vi "SHI_MCC_interface.vi"() -> ()   [LabVIEW 2017]
uses:
  <vilib>/httpClient/LabVIEWHTTPClient.lvlib
  <vilib>/httpClient/ClientHandle.ctl
  <vilib>/httpClient/POSTBuffer.vi
  msg7171_linux.llb/send single message.vi
  Type_Defs/Digital_Out.ctl
  Type_Defs/Digital_In_1.ctl
  Type_Defs/Analog_In.ctl
  msg7171_linux.llb/send multiple messages.vi
panel:
  out "Get Params json":string
  out "Get Status json":string
  in  "exit":bool
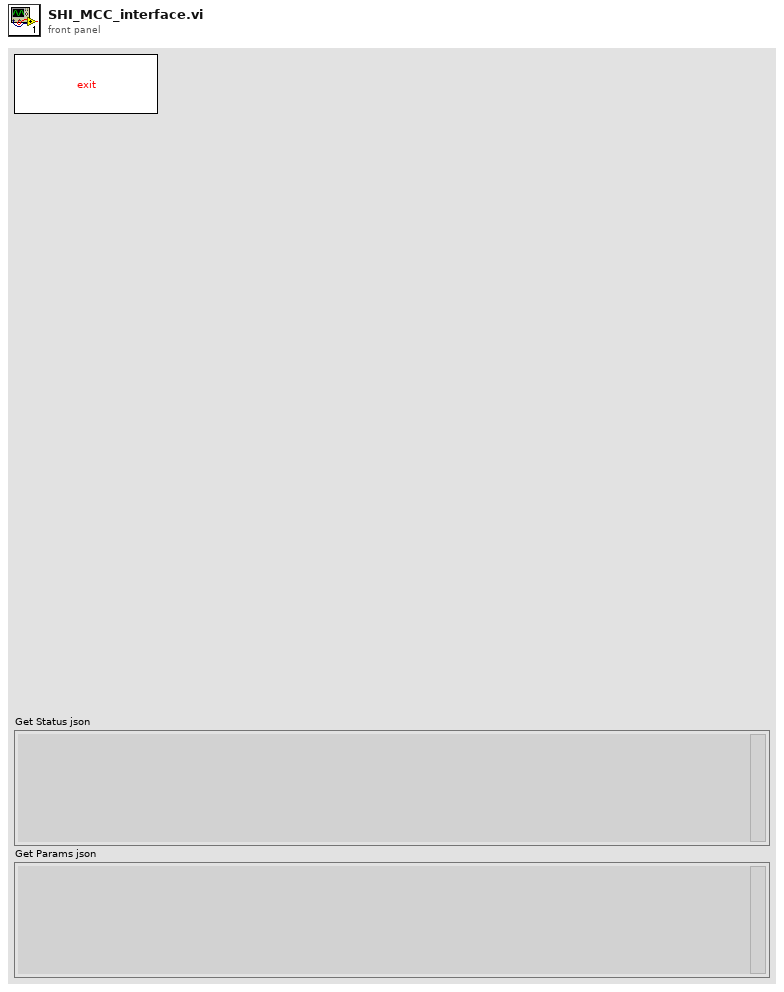
[diagram p1: front panel]
types:
  T1 = typedef "LabVIEWHTTPClient.lvlib/ClientHandle.ctl" = refnum<k1>
  T2 = cluster{"go":bool, "Http session":T1, "URL prefex":string, "Next get param":u32}
  T3 = typedef "Digital_Out.ctl" = cluster{"LN2-P EN":bool, "LN2-S EN":bool, "LN2-Sol EN":bool, "IR Lamp 1":bool, "IR Lamp 2":bool, "IR Lamp 3":bool, "IR Lamp 4":bool, "IR Lamp 5":bool, "IR Lamp 6":bool, "IR Lamp 7":bool, "IR Lamp 8":bool, "IR Lamp 9":bool, "IR Lamp 10":bool, "IR Lamp 11":bool, "IR Lamp 12":bool, "IR Lamp 13":bool, "IR Lamp 14":bool, "IR Lamp 15":bool, "IR Lamp 16":bool, "Heater SSR 1":bool, "Heater SSR 2":bool, "Heater SSR 3":bool, "Heater SSR 4":bool, "Heater SSR 5":bool, "Heater SSR 6":bool, "Heater SSR 7":bool, "Heater SSR 8":bool, "Heater SSR 9":bool, "Heater SSR 10":bool, "Heater SSR 11":bool, "Heater SSR 12":bool, "Heater SSR 13":bool, "Heater SSR 14":bool, "Heater SSR 15":bool, "Heater SSR 16":bool, "Heater SSR 17":bool, "Heater SSR 18":bool, "Heater SSR 19":bool, "Heater SSR 20":bool, "Heater SSR 21":bool, "MCC Power":bool, "MCC2 Power":bool, "RoughP GateValve":bool, "RoughP Start":bool, "CryoP GateValve":bool, "RoughP PurgeGass":bool, "LN2-S Sol":bool, "LN2-P Sol":bool, "CryoP Pwr Relay 1":bool, "CryoP Pwr Relay 2":bool, "RoughP Pwr Relay":bool}
  T4 = typedef "Digital_In_1.ctl" = cluster{"PG-SW-RoughP-Relay 1":bool, "PG-SW-RoughP-Relay 2":bool, "PG-SW-CryoP-Relay 1":bool, "PG-SW-CryoP-Relay 2":bool, "PG-SW-Chamber-Relay 1":bool, "PG-SW-Chamber-Relay 2":bool, "LN2-P-Sol-Open: NC":bool, "LN2-P-Sol-Open: O":bool, "LN2-P-Sol-Closed: NC":bool, "LN2-P-Sol-Closed: O":bool, "LN2-S-Sol-Open: NC":bool, "LN2-S-Sol-Open: O":bool, "LN2-S-Sol-Closed: NC":bool, "LN2-S-Sol-Closed: O":bool, "CryoP-GV-Open: NC":bool, "CryoP-GV-Open: O":bool, "CryoP-GV-Closed: NC":bool, "CryoP-GV-Closed: O":bool, "RoughP-GV-Open":bool, "RoughP-GV-Closed":bool, "RoughP-Pwr: NC":bool, "RoughP-Pwr: O":bool, "RoughP-On: NC":bool, "RoughP-On: O":bool, "Air supply LN2 OK":bool, "Air supply OK":bool}
  T5 = typedef "Analog_In.ctl" = cluster{"Cabinet Temp 1":u16, "Cabinet Temp 2":u16, "Cabinet Temp 3":u16, "fs Front Door 1":u16, "fs Front Door 2":u16, "fs Front Door 3":u16, "fs Back Door 1":u16, "fs Back Door 2":u16, "fs Back Door 3":u16, "Rough Pump Temp":u16, "pg Chamber":u16, "pg Cryo Pump":u16, "pg Rough Pump":u16, "LN2 platen":u16, "LN2 shroud":u16}
  T6 = cluster{"out":cluster{"LN2 Platen":u16, "LN2 Shroud":u16}, "in":T5}
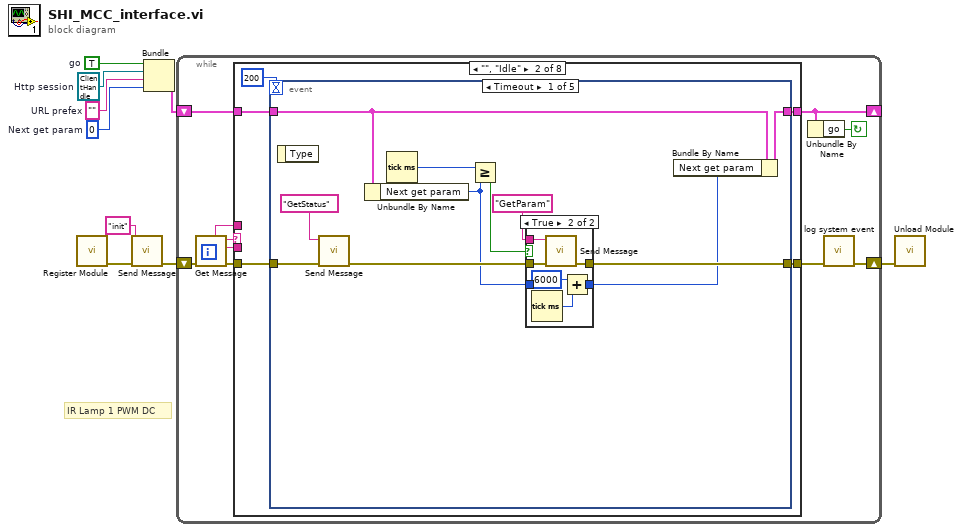
[diagram p0: block diagram]
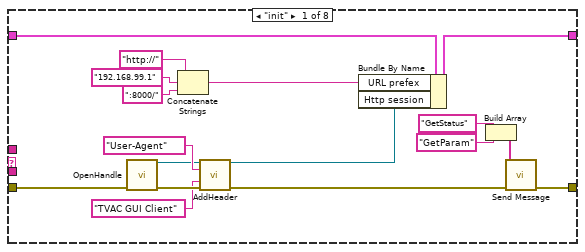
[diagram p2: hidden frame]
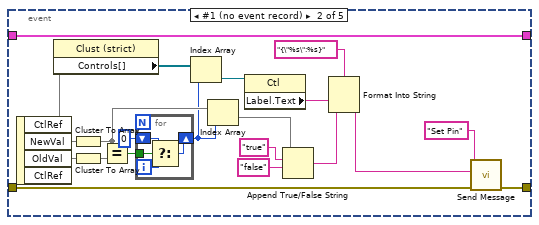
[diagram p4: hidden frame]
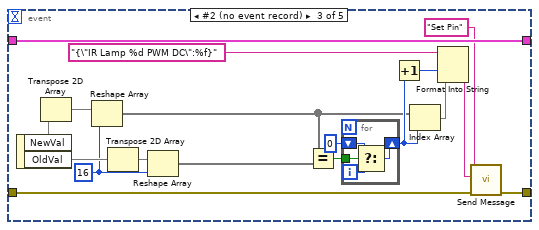
[diagram p5: hidden frame]
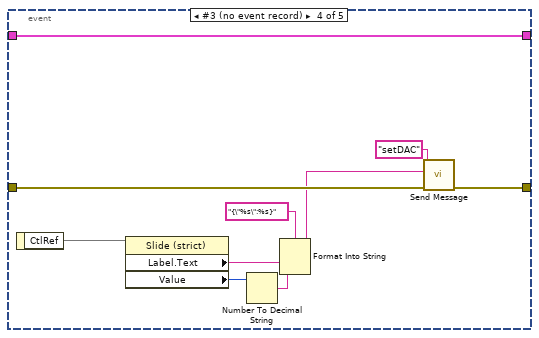
[diagram p6: hidden frame]
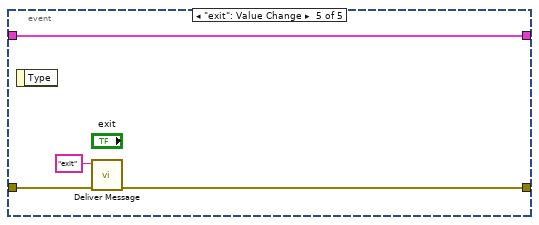
[diagram p7: hidden frame]
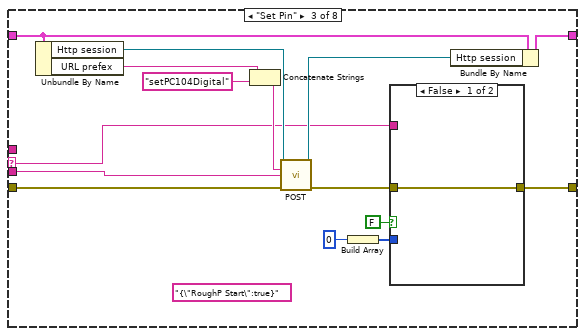
[diagram p8: hidden frame]
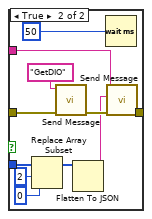
[diagram p9: hidden frame]
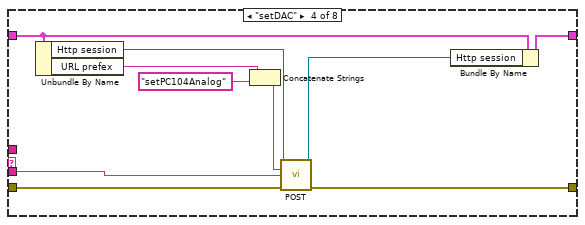
[diagram p10: hidden frame]
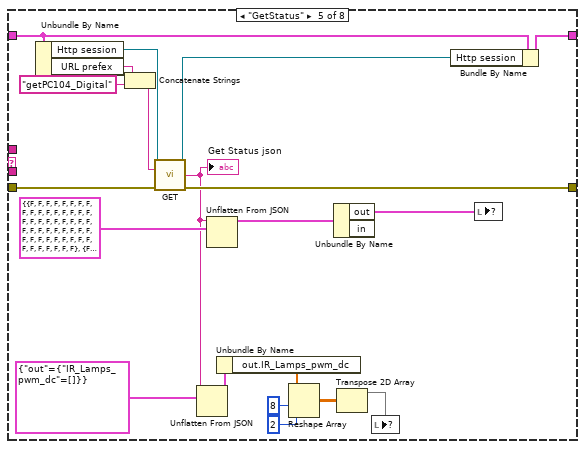
[diagram p11: hidden frame]
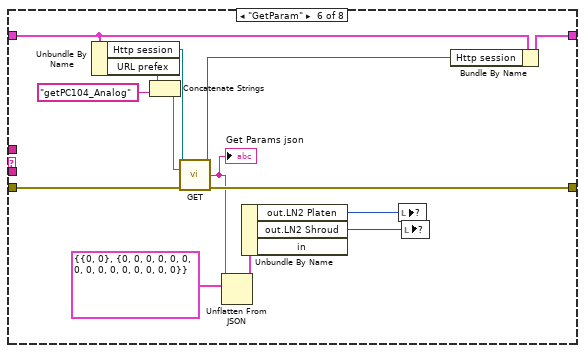
[diagram p12: hidden frame]
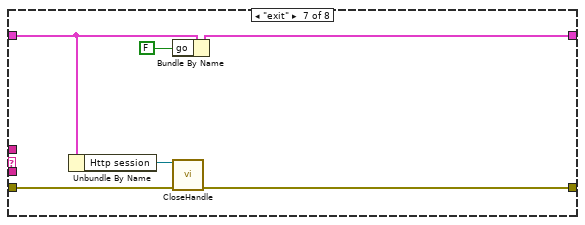
[diagram p13: hidden frame]
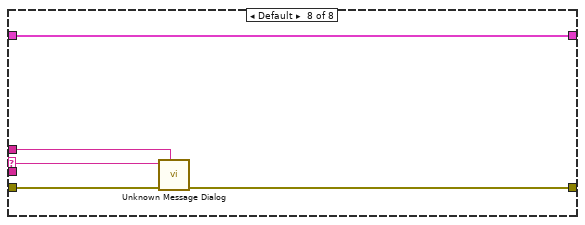
[diagram p14: hidden frame]
diagram:
  w1 = u32 0  # Next get param
  w5 = ""  # URL prefex
  w6 = T1 refnum  # Http session
  w7 = TRUE  # go
  # "IR Lamp 1 PWM DC"
  n1 = call "Register Module.vi"() -> ("error out"=w3:errorcluster)  [unwired: 10 in, 1 out]
  n2 = call-poly "Send Message.vi"("error in (no error)"=w3, "event"="init") -> ("error out"=w2:errorcluster)  [unwired: 9 in]
  n3 = Bundle("go"=w7, "Http session"=w6, "URL prefex"=w5, "Next get param"=w1) -> (w9:T2)  [unwired: 1 in]
  n4 = while {
    shift-left: w9 -> [w16]
    shift-right: [w13] -> _
    shift-right: [w11] -> w8
    shift-left: w2 -> [w19]
    stop <- w12 continue-if-true
    n5 = call "Get Message.vi"("error in (no error)"=w19) -> ("error out"=w17:errorcluster, "event buffer"=w18:string, "event"=w15:string, "source"=w14:string)  [unwired: 7 in]
    n6 = case shown="\"\", \"Idle\"" w15 {
      selector: w15 -> [_ _ w127 _ _ _ _ w203]
      tunnel: [w27 w38 w131 w153 w172 w187 w200 w205] -> w13
      tunnel: w16 -> [w36 w37 w130 w152 w171 w186 w195 w205]
      tunnel: w18 -> [_ _ w125 w149 _ _ _ _]
      tunnel: w17 -> [w31 w39 w129 w151 w174 w189 w198 w204]
      tunnel: w14 -> [_ _ _ _ _ _ _ w202]
      tunnel: [w23 w41 w128 w150 w173 w188 w197 w201] -> w10
      frame "init" {
        n7 = call <vilib>:"OpenHandle.vi"("error in (no error)"=w31) -> ("client handle out"=w32:T1, "error out"=w35:errorcluster)  [unwired: 13 in]
        n8 = Concatenate Strings("http://" ("url"), "192.168.99.1" ("Address"), ":8000/" ("url")) -> (w26:string)
        n9 = call <vilib>:"AddHeader.vi"("client handle"=w32, "header"="User-Agent", "value"="TVAC GUI Client", "error in (no error)"=w35) -> ("client handle out"=w25:T1, "error out"=w24:errorcluster)  [unwired: 10 in]
        n10 = Bundle By Name(cluster=w36, "URL prefex"=w26, "Http session"=w25) -> (w27:T2)
        n11 = Build Array("GetStatus" ("event"), "GetParam" ("event")) -> (w21:string[])
        n12 = call-poly "Send Message.vi"("error in (no error)"=w24, "event"=w21) -> ("error out"=w23:errorcluster)  [unwired: 9 in]
      }
      frame "", "Idle" {
        n13 = event shown="[0] Timeout" {
          selector: _ -> [_ _ _ _ _]
          dyn-events: _ -> [_ _ _ _ _]
          timeout: 200 ("milliseconds to wait") -> [_ _ _ _ _]
          tunnel: w39 -> [w52 w76 w100 w115 w121]
          tunnel: [w48 w75 w99 w116 w120] -> w41
          tunnel: [w44 w81 w103 w108 w118] -> w38
          tunnel: w37 -> [w47 w81 w103 w108 w118]
          event Timeout {
            n14 = event-data() -> ()  [unwired: 1 in, 1 out]
            n15 = call-poly "Send Message.vi"("error in (no error)"=w52, "event"="GetStatus") -> ("error out"=w50:errorcluster)  [unwired: 9 in]
            n16 = Unbundle By Name(w47) -> ("Next get param"=w42:u32)
            n17 = Tick Count (ms)() -> (millisecond timer value=w46:u32)
            n18 = Greater Or Equal?(x=w46, y=w42) -> (x >= y?=w45:bool)
            n19 = case shown="True" w45 {
              tunnel: w50 -> [w54 w60]
              tunnel: [w54 w59] -> w48
              tunnel: "GetParam" ("event") -> [_ w58]
              tunnel: [w53 w55] -> w43
              tunnel: w42 -> [w53 _]
              frame False {
              }
              frame True {
                n20 = Tick Count (ms)() -> (millisecond timer value=w57:u32)
                n21 = call-poly "Send Message.vi"("error in (no error)"=w60, "event"=w58) -> ("error out"=w59:errorcluster)  [unwired: 9 in]
                n22 = Add(x=u32 6000, y=w57) -> (x+y=w55:u32)
              }
            }
            n23 = Bundle By Name(cluster=w47, "Next get param"=w43) -> (w44:T2)
          }
          event #1 (no event record) {
            n24 = event-data() -> ("CtlRef"=w62, "NewVal"=w77, "OldVal"=w80)  [unwired: 1 in, 1 out]
            n25 = property class="Clust (strict)"(reference=w62) -> ("Controls[]"=w72:refnum<vi>[])  [unwired: 1 in, 2 out]
            n26 = Cluster To Array(cluster=w77) -> (array=w73:void[])
            n27 = Cluster To Array(cluster=w80) -> (array=w74:void[])
            n28 = Equal?(x=w73, y=w74) -> (x = y?=w79:bool)
            n29 = for {
              tunnel: w79 -> [w85]
              shift-right: [w84] -> w71
              shift-left: 0 -> [w83]
              i -> [w82]
              n30 = Select(t=w83, s=w85, f=w82) -> (s? t:f=w84:i32)
            }
            n31 = Index Array(array=w72, index=w71) -> (element=w70:refnum<vi>)
            n32 = Index Array(array=w73, index=w71) -> (element=w68)
            n33 = property class="Ctl"(reference=w70) -> ("Label.Text"=w65:string)  [unwired: 1 in, 2 out]
            n34 = Append True/False String(1:w68, 2:"false" ("false string"), 3:"true" ("true string")) -> (0:w63:string)  [unwired: 1 in]
            n35 = Format Into String(format string="{\"%s\":%s}" ("string"), w65, w63) -> (resulting string=w61:string)  [unwired: 2 in, 1 out]
            n36 = call-poly "Send Message.vi"("error in (no error)"=w76, "event buffer"=w61, "event"="Set Pin") -> ("error out"=w75:errorcluster)  [unwired: 8 in]
          }
          event #2 (no event record) {
            w88 = 16 ("dimension size")
            n37 = event-data() -> ("NewVal"=w93, "OldVal"=w90)  [unwired: 1 in]
            n38 = Transpose 2D Array(2D array=w93) -> (transposed array=w94:void[][])
            n39 = Reshape Array(w94, w88) -> (w92:void[])
            n40 = Transpose 2D Array(2D array=w90) -> (transposed array=w91:void[][])
            n41 = Reshape Array(w91, w88) -> (w89:void[])
            n42 = Equal?(x=w92, y=w89) -> (x = y?=w102:bool)
            n43 = for {
              tunnel: w102 -> [w107]
              shift-right: [w106] -> w95
              shift-left: 0 -> [w105]
              i -> [w104]
              n44 = Select(t=w105, s=w107, f=w104) -> (s? t:f=w106:i32)
            }
            n45 = Increment(x=w95) -> (x+1=w86:i32)
            n46 = Index Array(array=w92, index=w95) -> (element=w87)
            n47 = Format Into String(format string="{\"IR Lamp %d PWM DC\":%f}" ("string"), w86, w87) -> (resulting string=w96:string)  [unwired: 2 in, 1 out]
            n48 = call-poly "Send Message.vi"("error in (no error)"=w100, "event buffer"=w96, "event"="Set Pin") -> ("error out"=w99:errorcluster)  [unwired: 8 in]
          }
          event #3 (no event record) {
            n49 = event-data() -> ("CtlRef"=w114)  [unwired: 1 in]
            n50 = property class="Slide (strict)"(reference=w114) -> ("Label.Text"=w112:string, "Value"=w111:u16)  [unwired: 1 in, 2 out]
            n51 = Number To Decimal String(number=w111) -> (decimal integer string=w110:string)  [unwired: 1 in]
            n52 = Format Into String(format string="{\"%s\":%s}" ("string"), w112, w110) -> (resulting string=w109:string)  [unwired: 2 in, 1 out]
            n53 = call-poly "Send Message.vi"("error in (no error)"=w115, "event buffer"=w109, "event"="setDAC") -> ("error out"=w116:errorcluster)  [unwired: 8 in]
          }
          event "exit": Value Change {
            n54 = event-data() -> ()  [unwired: 1 in, 1 out]
            n55 = call "Deliver Message.vi"("error in (no error)"=w121, "event"="exit") -> ("error out"=w120:errorcluster)  [unwired: 9 in]
          }
        }
      }
      frame "Set Pin" {
        (unwired) "{\"RoughP Start\":true}" ("string")
        n56 = Unbundle By Name(w130) -> ("Http session"=w135:T1, "URL prefex"=w133:string)
        n57 = Concatenate Strings(w133, "setPC104Digital" ("url")) -> (w134:string)
        n58 = call-poly <vilib>:"POST.vi"("client handle"=w135, "url"=w134, "buffer"=w125, "error in (no error)"=w129) -> ("client handle out"=w136:T1, "error out"=w126:errorcluster)  [unwired: 8 in, 2 out]
        n59 = Build Array(0) -> (w123:i32[])
        n60 = case shown="False" FALSE {
          tunnel: [w137 w148] -> w128
          tunnel: w127 -> [_ w147]
          tunnel: w126 -> [w137 w146]
          tunnel: w123 -> [_ w143]
          frame False {
          }
          frame True {
            n61 = Replace Array Subset(array=w143, new element=0 ("new element/subarray"), index=2) -> (w139:i32[])
            n62 = call-poly "Send Message.vi"("error in (no error)"=w146, "event"="GetDIO") -> ("error out"=w145:errorcluster)  [unwired: 9 in]
            n63 = Flatten To JSON(anything=w139) -> (JSON string=w140:string)  [unwired: 2 in, 1 out]
            n64 = Wait (ms)(milliseconds to wait=u32 50) -> ()  [unwired: 1 out]
            n65 = call-poly "Send Message.vi"("error in (no error)"=w145, "event buffer"=w140, "event"=w147) -> ("error out"=w148:errorcluster)  [unwired: 8 in]
          }
        }
        n66 = Bundle By Name(cluster=w130, "Http session"=w136) -> (w131:T2)
      }
      frame "setDAC" {
        n67 = Unbundle By Name(w152) -> ("Http session"=w157:T1, "URL prefex"=w155:string)
        n68 = Concatenate Strings(w155, "setPC104Analog" ("url")) -> (w156:string)
        n69 = call-poly <vilib>:"POST.vi"("client handle"=w157, "url"=w156, "buffer"=w149, "error in (no error)"=w151) -> ("client handle out"=w158:T1, "error out"=w150:errorcluster)  [unwired: 8 in, 2 out]
        n70 = Bundle By Name(cluster=w152, "Http session"=w158) -> (w153:T2)
      }
      frame "GetStatus" {
        n71 = Unbundle By Name(w171) -> ("Http session"=w178:T1, "URL prefex"=w176:string)
        n72 = Concatenate Strings(w176, "getPC104_Digital" ("url")) -> (w177:string)
        n73 = call <vilib>:"GET.vi"("client handle"=w178, "url"=w177, "error in (no error)"=w174) -> ("client handle out"=w179:T1, "body"=w159:string, "error out"=w173:errorcluster)  [unwired: 9 in, 1 out]
        "Get Status json" <- w159
        n74 = Unflatten From JSON(JSON string=w159, type and defaults=cluster{"out":cluster{"IR_Lamps_pwm_dc":dbl[]}} {"out"={"IR_Lamps_pwm_dc"=[]}}) -> (value=w161:cluster{"out":cluster{"IR_Lamps_pwm_dc":dbl[]}})  [unwired: 5 in, 1 out]
        n75 = Unflatten From JSON(JSON string=w159, type and defaults=cluster{"out":T3, "in":T4} {"out"={"LN2-P EN"=FALSE, "LN2-S EN"=FALSE, "LN2-Sol EN"=FALSE, "IR Lamp 1"=FALSE, "IR Lamp 2"=FALSE, "IR Lamp 3"=FALSE, "IR Lamp 4"=FALSE, "IR Lamp 5"=FALSE, "IR Lamp 6"=FALSE, "IR Lamp 7"=FALSE, "IR Lamp 8"=FALSE, "IR Lamp 9"=FALSE, "IR Lamp 10"=FALSE, "IR Lamp 11"=FALSE, "IR Lamp 12"=FALSE, "IR Lamp 13"=FALSE, "IR Lamp 14"=FALSE, "IR Lamp 15"=FALSE, "IR Lamp 16"=FALSE, "Heater SSR 1"=FALSE, "Heater SSR 2"=FALSE, "Heater SSR 3"=FALSE, "Heater SSR 4"=FALSE, "Heater SSR 5"=FALSE, "Heater SSR 6"=FALSE, "Heater SSR 7"=FALSE, "Heater SSR 8"=FALSE, "Heater SSR 9"=FALSE, "Heater SSR 10"=FALSE, "Heater SSR 11"=FALSE, "Heater SSR 12"=FALSE, "Heater SSR 13"=FALSE, "Heater SSR 14"=FALSE, "Heater SSR 15"=FALSE, "Heater SSR 16"=FALSE, "Heater SSR 17"=FALSE, "Heater SSR 18"=FALSE, "Heater SSR 19"=FALSE, "Heater SSR 20"=FALSE, "Heater SSR 21"=FALSE, "MCC Power"=FALSE, "MCC2 Power"=FALSE, "RoughP GateValve"=FALSE, "RoughP Start"=FALSE, "CryoP GateValve"=FALSE, "RoughP PurgeGass"=FALSE, "LN2-S Sol"=FALSE, "LN2-P Sol"=FALSE, "CryoP Pwr Relay 1"=FALSE, "CryoP Pwr Relay 2"=FALSE, "RoughP Pwr Relay"=FALSE}, "in"={"PG-SW-RoughP-Relay 1"=FALSE, "PG-SW-RoughP-Relay 2"=FALSE, "PG-SW-CryoP-Relay 1"=FALSE, "PG-SW-CryoP-Relay 2"=FALSE, "PG-SW-Chamber-Relay 1"=FALSE, "PG-SW-Chamber-Relay 2"=FALSE, "LN2-P-Sol-Open: NC"=FALSE, "LN2-P-Sol-Open: O"=FALSE, "LN2-P-Sol-Closed: NC"=FALSE, "LN2-P-Sol-Closed: O"=FALSE, "LN2-S-Sol-Open: NC"=FALSE, "LN2-S-Sol-Open: O"=FALSE, "LN2-S-Sol-Closed: NC"=FALSE, "LN2-S-Sol-Closed: O"=FALSE, "CryoP-GV-Open: NC"=FALSE, "CryoP-GV-Open: O"=FALSE, "CryoP-GV-Closed: NC"=FALSE, "CryoP-GV-Closed: O"=FALSE, "RoughP-GV-Open"=FALSE, "RoughP-GV-Closed"=FALSE, "RoughP-Pwr: NC"=FALSE, "RoughP-Pwr: O"=FALSE, "RoughP-On: NC"=FALSE, "RoughP-On: O"=FALSE, "Air supply LN2 OK"=FALSE, "Air supply OK"=FALSE}}) -> (value=w167:cluster{"out":T3, "in":T4})  [unwired: 5 in, 1 out]
        n76 = Unbundle By Name(w161) -> ("out.IR_Lamps_pwm_dc"=w160:dbl[])
        n77 = Reshape Array(w160, 8 ("dimension size"), 2 ("dimension size")) -> (w164:dbl[][])
        n78 = Unbundle By Name(w167) -> ("out"=w170:T3, "in"=w169:T4)
        n79 = Transpose 2D Array(2D array=w164) -> (transposed array=w163:dbl[][])
        n80 = local write item#-1(w163) -> ()
        n81 = Bundle By Name(cluster=w171, "Http session"=w179) -> (w172:T2)
        n82 = local write item#-1(w170) -> ()
      }
      frame "GetParam" {
        n83 = Unbundle By Name(w186) -> ("Http session"=w193:T1, "URL prefex"=w191:string)
        n84 = Concatenate Strings(w191, "getPC104_Analog" ("url")) -> (w192:string)
        n85 = call <vilib>:"GET.vi"("client handle"=w193, "url"=w192, "error in (no error)"=w189) -> ("client handle out"=w194:T1, "body"=w181:string, "error out"=w188:errorcluster)  [unwired: 9 in, 1 out]
        "Get Params json" <- w181
        n86 = Unflatten From JSON(JSON string=w181, type and defaults=T6 {"out"={"LN2 Platen"=0, "LN2 Shroud"=0}, "in"={"Cabinet Temp 1"=0, "Cabinet Temp 2"=0, "Cabinet Temp 3"=0, "fs Front Door 1"=0, "fs Front Door 2"=0, "fs Front Door 3"=0, "fs Back Door 1"=0, "fs Back Door 2"=0, "fs Back Door 3"=0, "Rough Pump Temp"=0, "pg Chamber"=0, "pg Cryo Pump"=0, "pg Rough Pump"=0, "LN2 platen"=0, "LN2 shroud"=0}}) -> (value=w184:T6)  [unwired: 5 in, 1 out]
        n87 = Unbundle By Name(w184) -> ("out.LN2 Platen"=w183:u16, "out.LN2 Shroud"=w182:u16, "in"=w180:T5)
        n88 = local write item#-1(w183) -> ()
        n89 = local write item#-1(w182) -> ()
        n90 = Bundle By Name(cluster=w186, "Http session"=w194) -> (w187:T2)
      }
      frame "exit" {
        n91 = Unbundle By Name(w195) -> ("Http session"=w196:T1)
        n92 = Bundle By Name(cluster=w195, "go"=FALSE ("Bundle Element")) -> (w200:T2)
        n93 = call <vilib>:"CloseHandle.vi"("client handle"=w196, "error in (no error)"=w198) -> ("error out"=w197:errorcluster)  [unwired: 13 in]
      }
      frame Default {
        n94 = call "Unknown Message Dialog.vi"("source"=w202, "error in (no error)"=w204, "event name"=w203) -> ("error out"=w201:errorcluster)  [unwired: 8 in]
      }
    }
    n95 = Unbundle By Name(w13) -> ("go"=w12:bool)
    n96 = call "log system event.vi"("error in (no error)"=w10) -> ("error out"=w11:errorcluster)  [unwired: 9 in, 1 out]
  }
  n97 = call "Unload Module.vi"("error in (no error)"=w8) -> ()  [unwired: 10 in, 1 out]
